vi "Wait-for-message.vi"(8 "error in (no error)":errorcluster, 9 "Timeout":i32=5000 caption="Timeout [ms]", 11 "ModComm in":T1) -> (0 "error out":errorcluster, 1 "New message?":bool, 2 "Message":refnum<class "Message.lvclass">, 3 "ModComm out":T1)   [LabVIEW 2013, in "Server.lvlib" / "Server.lvclass"]
uses:
  Server.lvclass
  Object-reference.ctl
  Messages/Sources/Message.lvclass
  Server.lvclass/Server.ctl
  Read Server channel.vi
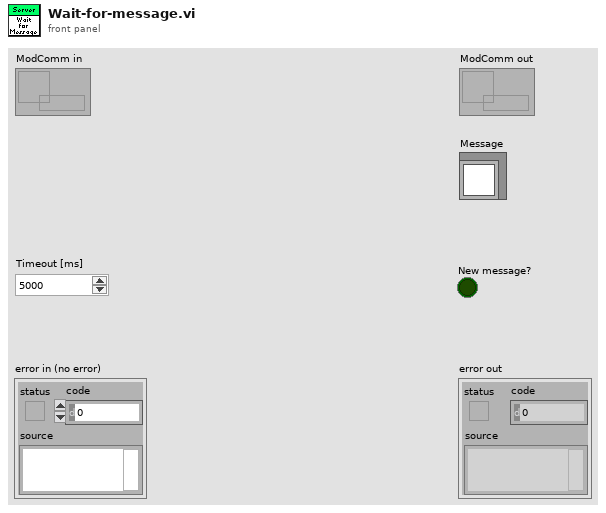
[diagram p1: front panel]
types:
  T1 = typedef "Server.lvlib/Server.lvclass/Object-reference.ctl" = refnum<data-value>
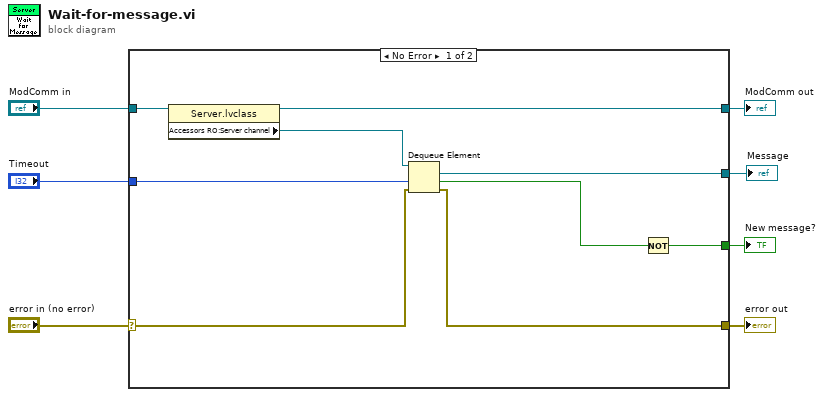
[diagram p0: block diagram]
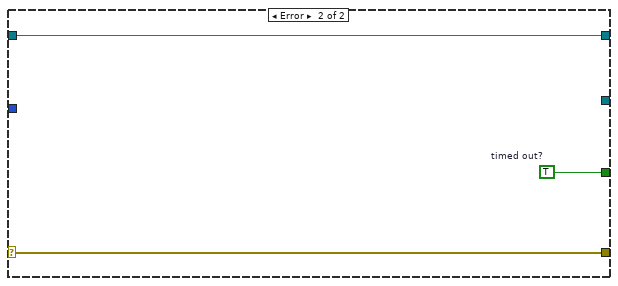
[diagram p2: hidden frame]
diagram:
  n1 = case shown="No Error" "error in (no error)" {
    selector: "error in (no error)" -> [w13 w19]
    tunnel: [w12 w19] -> w6
    tunnel: [w15 w18] -> w4
    tunnel: "ModComm in" -> [w16 w18]
    tunnel: "Timeout" -> [w14 _]
    tunnel: [w8 w17] -> w2
    tunnel: [w9 _] -> w1
    frame No Error {
      n2 = property class="Server.lvclass"(reference=w16) -> (reference out=w15:T1, "Accessors RO:Server channel"=w11:refnum<queue>)  [unwired: 1 in, 1 out]
      n3 = Dequeue Element(queue=w11, timeout in ms (-1)=w14, error in (no error)=w13) -> (element=w9:refnum<class "Message.lvclass">, timed out?=w10:bool, error out=w12:errorcluster)  [unwired: 1 out]
      n4 = Not(x=w10) -> (.not. x?=w8:bool)
    }
    frame Error {
      w17 = TRUE  # timed out?
    }
  }
  "error out" <- w6
  "ModComm out" <- w4
  "New message?" <- w2
  "Message" <- w1
